vi "Autonomous Independent.vi"   [LabVIEW 2013]
doc: "This VI is called when autonomous begins, and will automatically be terminated when autonomous ends. You can carry out timed or sensor driven robot movement independently without needing to return to the caller."
uses:
  <vilib>/Rock Robotics/WPI/Solenoid/WPI_SolenoidValue.ctl
  <vilib>/Rock Robotics/WPI/RobotDrive/WPI_RobotDriveGetSetRefNum.vi
  <vilib>/Rock Robotics/WPI/Solenoid/Deprecated/WPI_SolenoidGetBool.vi
  <vilib>/Rock Robotics/WPI/Solenoid/WPI_SolenoidSetEnum.vi
panel:
  # "Be sure to right-click and choose Data Operations>>Make Current Value default if you want to save the array values with the VI"
types:
  T1 = typedef "WPI_RobotDriveDevRef.ctl" = cluster{"DevStatus":errorcluster, "Motors[]":T2[], "Square Inputs":bool, "Max Output":dbl, "Isochronous":bool}
  T2 = typedef "WPI_MotorControlDeviceRef.ctl" = cluster{"DeviceStatus":errorcluster, "Type":enum16{"PWM", "CAN"}, "PWM":cluster{"Digital Module":T3, "PWM Channel":T4, "DeadBand":T5}, "CAN":cluster{"Device Number":u8, "Control Mode":T6, "Semaphore":T7, "Max Vout":dbl}, "Invert":bool, "TransformRef":T8, "InvTransformRef":T8}
  T3 = typedef "FPGA_TypedefDigitalModule.ctl" = enum16{"Digital Module 1", "Digital Module 2"}
  T4 = typedef "FPGA_DIOPWMChannel.ctl" = enum8{"PWM 1", "PWM 2", "PWM 3", "PWM 4", "PWM 5", "PWM 6", "PWM 7", "PWM 8", "PWM 9", "PWM 10", "Invalid"}
  T5 = typedef "WPI_PWMDeadband.ctl" = cluster{"Name":string, "maxPositivePwm":i32, "minPositivePwm":i32, "centerPwm":i32, "maxNegativePwm":i32, "minNegativePwm":i32, "angularRange":u16}
  T6 = typedef "WPI_CANJaguar_ControlMode.ctl" = enum8{"Percent VBus", "Current", "Speed", "Position", "Voltage"}
  T7 = typedef "Semaphore RefNum" = refnum<k1>
  T8 = typedef "WPI_PWMTransform_ConPane.ctl" = refnum<vi>
  T9 = typedef "WPI_SolenoidDevRef.ctl" = cluster{"DevStatus":errorcluster, "Solenoid Module":T10, "Forward Solenoid Channel":T11, "Reverse Solenoid Channel":T11}
  T10 = typedef "FPGA_TypedefSolenoidModule.ctl" = enum16{"Solenoid Module 1", "Solenoid Module 2"}
  T11 = typedef "WPI_SolenoidChannel.ctl" = enum8{"Solenoid 1", "Solenoid 2", "Solenoid 3", "Solenoid 4", "Solenoid 5", "Solenoid 6", "Solenoid 7", "Solenoid 8", "Invalid"}
  T12 = typedef "WPI_SolenoidValue.ctl" = enum16{"Off", "On", "Forward", "Reverse"}
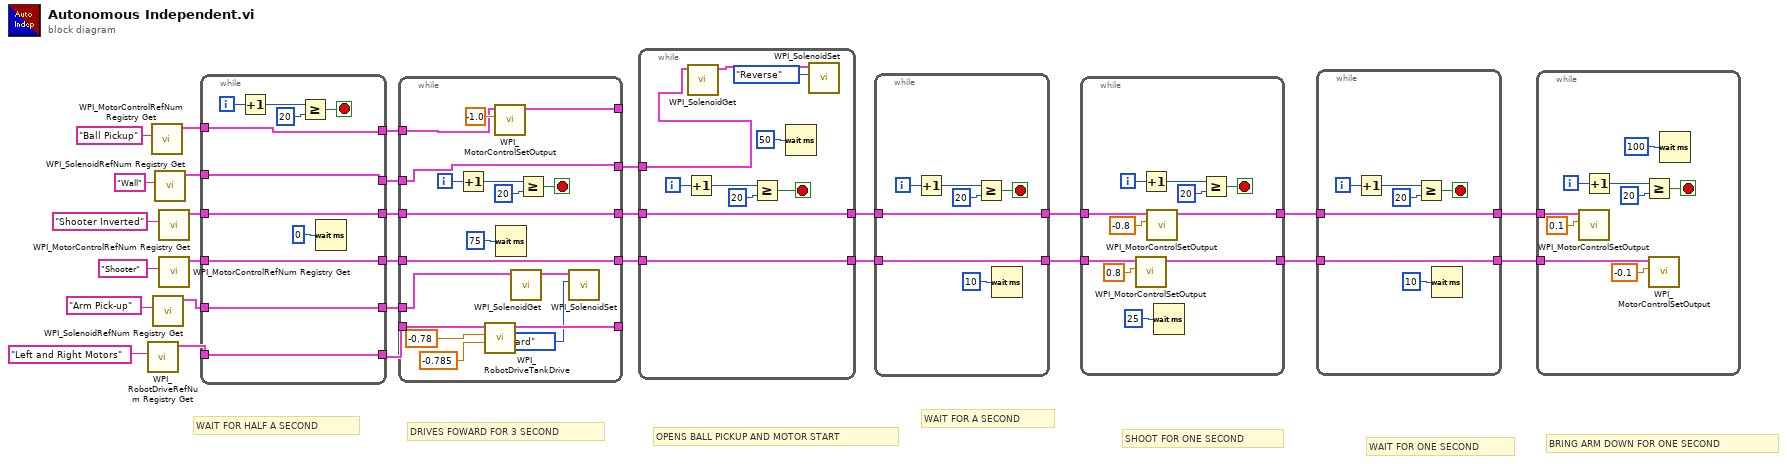
[diagram p0: block diagram]
diagram:
  # "WAIT FOR A SECOND"
  # "WAIT FOR ONE SECOND"
  # "BRING ARM DOWN FOR ONE SECOND"
  # "WAIT FOR HALF A SECOND"
  # "SHOOT FOR ONE SECOND"
  # "OPENS BALL PICKUP AND MOTOR START"
  # "DRIVES FOWARD FOR 3 SECOND"
  n1 = call <vilib>:"WPI_RobotDriveRefNum Registry Get.vi"("refnum name"="Left and Right Motors") -> ("RobotDriveDevRef"=w26:T1)  [unwired: 9 in, 1 out]
  n2 = call <vilib>:"WPI_MotorControlRefNum Registry Get.vi"("refnum name"="Ball Pickup") -> ("MotorControlDevRef"=w2:T2)  [unwired: 9 in, 1 out]
  n3 = call <vilib>:"WPI_SolenoidRefNum Registry Get.vi"("refnum name"="Arm Pick-up") -> ("SolenoidDevRef"=w27:T9)  [unwired: 9 in, 1 out]
  n4 = call <vilib>:"WPI_SolenoidRefNum Registry Get.vi"("refnum name"="Wall") -> ("SolenoidDevRef"=w6:T9)  [unwired: 9 in, 1 out]
  n5 = call <vilib>:"WPI_MotorControlRefNum Registry Get.vi"("refnum name"="Shooter Inverted") -> ("MotorControlDevRef"=w23:T2)  [unwired: 9 in, 1 out]
  n6 = call <vilib>:"WPI_MotorControlRefNum Registry Get.vi"("refnum name"="Shooter") -> ("MotorControlDevRef"=w22:T2)  [unwired: 9 in, 1 out]
  n7 = while {
    tunnel: w27 -> [w32]
    tunnel: [w40] -> w8
    tunnel: w26 -> [w40]
    tunnel: w23 -> [w34]
    tunnel: [w34] -> w20
    tunnel: w22 -> [w33]
    tunnel: [w33] -> w21
    tunnel: [w32] -> w17
    tunnel: [w31] -> w5
    tunnel: w6 -> [w31]
    tunnel: [w30] -> w1
    tunnel: w2 -> [w30]
    i -> [w37]
    stop <- w36 stop-if-true
    n8 = Increment(x=w37) -> (x+1=w38:i32)
    n9 = Greater Or Equal?(x=w38, y=20) -> (x >= y?=w36:bool)
    n10 = Wait (ms)(milliseconds to wait=u32 0) -> ()  [unwired: 1 out]
  }
  n11 = while {
    tunnel: w8 -> [w58]
    tunnel: [w51] -> _
    tunnel: w20 -> [w49]
    tunnel: [w49] -> w19
    tunnel: w21 -> [w48]
    tunnel: [w48] -> w18
    tunnel: w17 -> [w44]
    tunnel: w5 -> [w47]
    tunnel: [w47] -> w4
    tunnel: w1 -> [w42]
    tunnel: [w41] -> _
    i -> [w56]
    stop <- w53 stop-if-true
    n12 = Increment(x=w56) -> (x+1=w55:i32)
    n13 = call <vilib>:"WPI_RobotDriveTankDrive.vi"("Right axis value"=-0.785 ("Y axis value"), "Left axis value"=-0.78 ("X axis value"), "RobotDriveDevRef"=w58) -> ("RobotDriveDevRef"=w51:T1)  [unwired: 6 in, 2 out]
    n14 = call <vilib>:"WPI_MotorControlSetOutput.vi"("Output"=-1.0, "MotorControlDevRef"=w42) -> ("MotorControlDevRef"=w41:T2)  [unwired: 7 in, 2 out]
    n15 = Wait (ms)(milliseconds to wait=u32 75) -> ()  [unwired: 1 out]
    n16 = call-poly <vilib>:"WPI_SolenoidGet.vi"("SolenoidDevRef"=w44) -> ("SolenoidDevRef"=w46:T9)  [unwired: 8 in, 2 out]
    n17 = Greater Or Equal?(x=w55, y=20) -> (x >= y?=w53:bool)
    n18 = call-poly <vilib>:"WPI_SolenoidSet.vi"("Value"=WPI_SolenoidValue."Forward", "SolenoidDevRef"=w46) -> ()  [unwired: 8 in, 2 out]
  }
  n19 = while {
    tunnel: [w68] -> w10
    tunnel: w19 -> [w68]
    tunnel: [w67] -> w11
    tunnel: w18 -> [w67]
    tunnel: w4 -> [w60]
    i -> [w65]
    stop <- w63 stop-if-true
    n20 = Increment(x=w65) -> (x+1=w66:i32)
    n21 = call-poly <vilib>:"WPI_SolenoidGet.vi"("SolenoidDevRef"=w60) -> ("SolenoidDevRef"=w61:T9)  [unwired: 8 in, 2 out]
    n22 = Greater Or Equal?(x=w66, y=20) -> (x >= y?=w63:bool)
    n23 = Wait (ms)(milliseconds to wait=u32 50) -> ()  [unwired: 1 out]
    n24 = call-poly <vilib>:"WPI_SolenoidSet.vi"("Value"=WPI_SolenoidValue."Reverse", "SolenoidDevRef"=w61) -> ()  [unwired: 8 in, 2 out]
  }
  n25 = while {
    tunnel: [w70] -> w12
    tunnel: w11 -> [w70]
    tunnel: w10 -> [w69]
    tunnel: [w69] -> w9
    i -> [w75]
    stop <- w72 stop-if-true
    n26 = Increment(x=w75) -> (x+1=w74:i32)
    n27 = Greater Or Equal?(x=w74, y=20) -> (x >= y?=w72:bool)
    n28 = Wait (ms)(milliseconds to wait=u32 10) -> ()  [unwired: 1 out]
  }
  n29 = while {
    tunnel: [w79] -> w16
    tunnel: [w78] -> w15
    tunnel: w12 -> [w77]
    tunnel: w9 -> [w76]
    i -> [w84]
    stop <- w83 stop-if-true
    n30 = call <vilib>:"WPI_MotorControlSetOutput.vi"("Output"=0.8, "MotorControlDevRef"=w77) -> ("MotorControlDevRef"=w78:T2)  [unwired: 7 in, 2 out]
    n31 = Increment(x=w84) -> (x+1=w86:i32)
    n32 = call <vilib>:"WPI_MotorControlSetOutput.vi"("Output"=-0.8, "MotorControlDevRef"=w76) -> ("MotorControlDevRef"=w79:T2)  [unwired: 7 in, 2 out]
    n33 = Wait (ms)(milliseconds to wait=u32 25) -> ()  [unwired: 1 out]
    n34 = Greater Or Equal?(x=w86, y=20) -> (x >= y?=w83:bool)
  }
  n35 = while {
    tunnel: [w88] -> w13
    tunnel: w16 -> [w88]
    tunnel: [w87] -> w14
    tunnel: w15 -> [w87]
    i -> [w91]
    stop <- w90 stop-if-true
    n36 = Increment(x=w91) -> (x+1=w93:i32)
    n37 = Greater Or Equal?(x=w93, y=20) -> (x >= y?=w90:bool)
    n38 = Wait (ms)(milliseconds to wait=u32 10) -> ()  [unwired: 1 out]
  }
  n39 = while {
    tunnel: w14 -> [w95]
    tunnel: w13 -> [w94]
    i -> [w100]
    stop <- w99 stop-if-true
    n40 = call <vilib>:"WPI_MotorControlSetOutput.vi"("Output"=0.1, "MotorControlDevRef"=w94) -> ()  [unwired: 7 in, 3 out]
    n41 = Increment(x=w100) -> (x+1=w101:i32)
    n42 = Greater Or Equal?(x=w101, y=20) -> (x >= y?=w99:bool)
    n43 = call <vilib>:"WPI_MotorControlSetOutput.vi"("Output"=-0.1, "MotorControlDevRef"=w95) -> ()  [unwired: 7 in, 3 out]
    n44 = Wait (ms)(milliseconds to wait=u32 100) -> ()  [unwired: 1 out]
  }
